vi "List All Menus.vi"(7 "menu reference":refnum<k9>, 8 "error in (no error)":errorcluster) -> (0 "error in (no error) (dup)":errorcluster, 2 "Array":string[](array[string]))   [LabVIEW 2017, in "TagDB RefManager.lvlib"]
uses:
  TagDB RefManager.lvlib
  <userlib>/_NEVSTOP/TagDB/TagDB.lvlib
panel:
  out "size(s)":i32
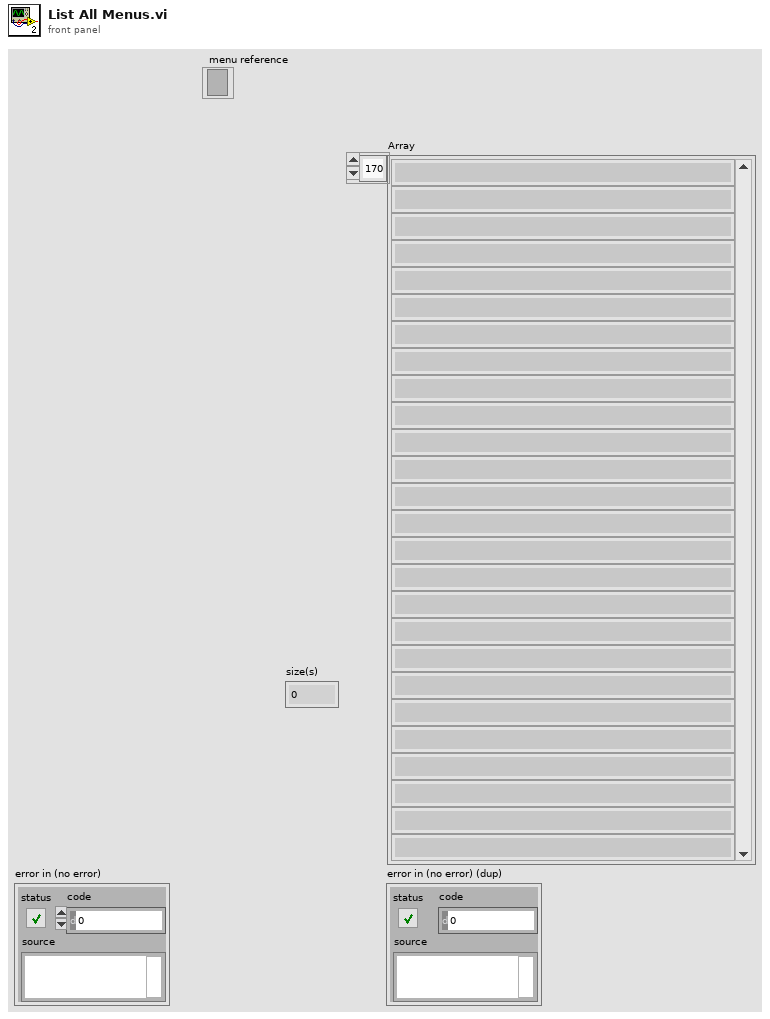
[diagram p1: front panel]
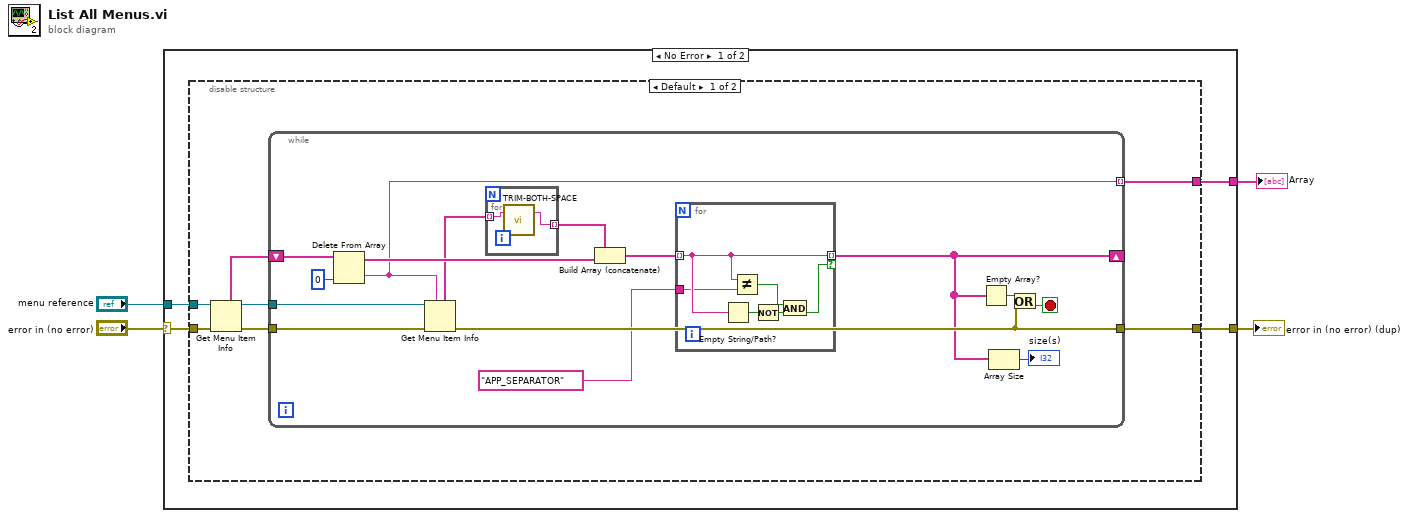
[diagram p0: block diagram]
diagram:
  n1 = case shown="No Error" "error in (no error)" {
    selector: "error in (no error)" -> [w7 w40]
    tunnel: "menu reference" -> [w8 _]
    tunnel: [w5 w40] -> w2
    tunnel: [w6 _] -> w1
    frame No Error {
      n2 = disable-structure shown="Default" {
        disable-tunnel: w8 -> [w12 _]
        disable-tunnel: w7 -> [w11 w39]
        disable-tunnel: [w10 _] -> w6
        disable-tunnel: [w9 w39] -> w5
        frame condition #0 (active) {
          n3 = Get Menu Item Info(8:w11, 11:w12) -> (0:w13:errorcluster, 3:w15:refnum<k9>, 5:w14:string[])  [unwired: 1 in, 4 out]
          n4 = while {
            tunnel: w15 -> [w30]
            shift-right: [w17] -> _
            shift-left: w14 -> [w29]
            tunnel: [w26] -> w10 mode=indexing
            tunnel: w13 -> [w22]
            tunnel: [w19] -> w9
            stop <- w21 stop-if-true
            n5 = Delete From Array(array=w29, index=0) -> (deleted portion=w26:string, array with subset deleted=w28:string[])  [unwired: 1 in]
            n6 = Get Menu Item Info(7:w26, 8:w22, 11:w30) -> (0:w19:errorcluster, 5:w27:string[])  [unwired: 5 out]
            n7 = for {
              tunnel: w27 -> [w38] mode=indexing
              tunnel: [w37] -> w23 mode=indexing
              n8 = call <userlib>:"TRIM-BOTH-SPACE.vi"("name in"=w38) -> ("name out"=w37:string)  [unwired: 2 in]
            }
            n9 = Build Array (concatenate)(w23, w28) -> (w18:string[])
            n10 = for {
              tunnel: w18 -> [w34] mode=indexing
              tunnel: [w34] -> w17 mode=indexing if=w32
              tunnel: "APP_SEPARATOR" -> [w33]
              n11 = Empty String/Path?(string/path=w34) -> (empty?=w36:bool)
              n12 = Not Equal?(x=w34, y=w33) -> (x != y?=w31:bool)
              n13 = Not(x=w36) -> (.not. x?=w35:bool)
              n14 = And(x=w31, y=w35) -> (x .and. y?=w32:bool)
            }
            n15 = Empty Array?(array=w17) -> (empty?=w20:bool)
            n16 = Array Size(array=w17) -> (size(s)=→"size(s)":i32)
            n17 = Or(x=w20, y=w19) -> (x .or. y?=w21:bool)
          }
        }
        frame condition #1 {
        }
      }
    }
    frame Error {
    }
  }
  "error in (no error) (dup)" <- w2
  "Array" <- w1
